vi "Walsh Hadamard Inverse PtByPt.vi"(2 "initialize":bool, 3 "sample length":i32=100, 5 "x":dbl format="%0.2f") -> (0 "error":i32, 1 "Walsh Hadamard Inverse {X}":dbl[](array[numeric]))   [LabVIEW 2020, in "NI_PtbyPt.lvlib"]
doc: "Performs the inverse of the real Walsh Hadamard transform."
uses:
  NI_PtbyPt.lvlib
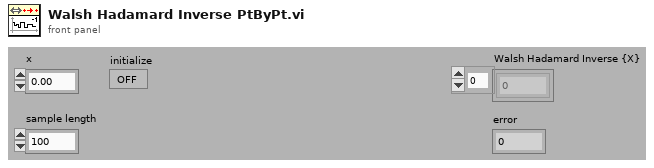
[diagram p1: front panel]
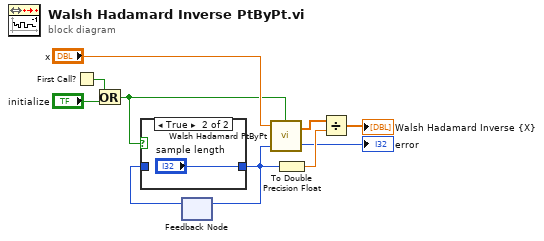
[diagram p0: block diagram]
diagram:
  n1 = First Call?() -> (First Call?: T/F=w7:bool)
  n2 = Or(x=w7, y="initialize") -> (x .or. y?=w3:bool)
  n3 = feedback #1() -> (w1:i32)  [unwired: 1 in]
  n4 = case shown="True" w3 {
    tunnel: [w11 "sample length"] -> w2
    tunnel: w1 -> [w11 _]
    frame False {
    }
    frame True {
    }
  }
  n5 = feedback-in #1(w2) -> ()
  n6 = call "Walsh Hadamard PtByPt.vi"("initialize"=w3, "sample length"=w2, "x"="x") -> ("error"=→"error":i32, "Walsh Hadamard {X}"=w4:dbl[])  [unwired: 1 in]
  n7 = To Double Precision Float(number=w2) -> (double precision float=w9:dbl)
  n8 = Divide(x=w4, y=w9) -> (x/y=→"Walsh Hadamard Inverse {X}":dbl[])
